vi "Lab Temp Monitor.vi"() -> ()   [LabVIEW 2012]
uses:
  Automated Dish Machine/LabVIEW/ADM2 - QMH Layout/support/Message Queue/Message Cluster.ctl
  <vilib>/Utility/error.llb/DialogType.ctl
  Automated Dish Machine/LabVIEW/ADM2 - QMH Layout/support/Message Queue/Message Queue.lvlib
panel:
  out "Limits":dbl[](array[numeric])
  in  "STOP":bool
  in  "Channel Names":string[](array[string])=["One", "Two", "Three", "Four", "Five", "Six"]
  out "Test Display":string
  in  "CONFIG":bool
  in  "Limit 1":dbl=52.0
  in  "Limit 2":dbl=56.0
  out "Timers":u32[](array[numeric])=[1, 95] format="%<%H:%M:%S>t"
  in  "Email / Image Rate":u32=7200 format="%<%H:%M:%S>t"
  in  "Graph / Log Rate":u32=2 format="%<%H:%M:%S>t"
  in  "START":bool
  in  "MAIN TAB":enum32{"Page 1", "Page 2"}(tab)
  out "Graph":cluster{"t0":dbl, "dx":dbl, "Y Values":dbl[][]}(graph)
  out "Email Error":errorcluster
  out "UI ERROR":errorcluster
  out "DAQ Error":errorcluster
  in  "9213 Config":T1={"Sample Rate [Hz]"=100.0, "Samples/Ch"=1, "Ch Used"=1, "Rolling Average"=1, "HI/LO Trim [%]"=1.0, "Sample Timing Engine"=2} {"Ch Used" min=1 max=16 step=1; "Sample Timing Engine" max=2; "Sample Rate [Hz]" min=0.0001 max=100.0 format="%#_6p"; "Samples/Ch" min=1 step=1; "Rolling Average" min=1 step=1; "HI/LO Trim [%]" min=1.0 max=99.0}
  in  "9213 Name":tag="cDAQ2Mod1"
  out "9213 Error":errorcluster
  in  "Image File Path":path=path "C:/Users/ottinbr/Documents/Projects/John Bolduc/Lab Temp Monitor/a.jpg"
  in  "Log Folder Path":path=path "C:/Users/ottinbr/Documents/Projects/John Bolduc/Lab Temp Monitor/a.jpg"
  out "MAIN Queue":T2
  out "MAIN Loop":i32
  out "EVENT Loop":i32
  out "DAQ Queue":T2
  out "DAQ Loop":i32
  out "Last Sent Time":timestamp format="%<%I:%M:%S %p\n%x>T"
  out "Image Error":errorcluster
  in  "EMAIL":bool
  in  "EXIT PROGRAM":bool
  in  "ECOLAB BUTTON":bool=TRUE
  out "Measurements":dbl[](array[numeric]) format="%.2f"
  # "F&B Lab Temp. Monitor"
  # "SETPOINT"
  # "ELAPSED"
  # "Temp Limits"
  # "Created by Blake Otting  June 2013"
  # "Last Updated 7-11-13"
  # "HH:MM:SS"
  # "°C"
  # "HH:MM:SS"
  # "°C"
  # "9213 Configuration"
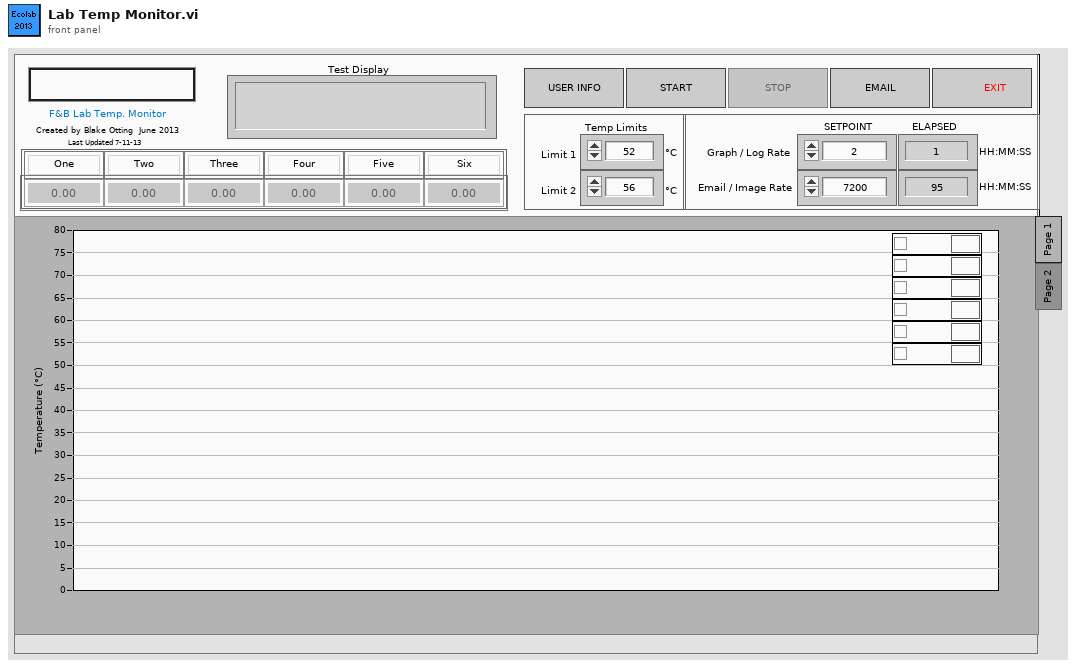
[diagram p1: front panel]
types:
  T1 = cluster{"Sample Rate [Hz]":dbl, "Samples/Ch":i32, "Ch Used":i32, "Rolling Average":i32, "HI/LO Trim [%]":dbl, "Sample Timing Engine":u32}
  T2 = cluster{"Message":string, "Message Data":variant}
  T3 = cluster{"Graph":cluster{"t0":dbl, "dx":dbl, "Y Values":dbl[][]}, "Image File Path":path, "Data Row":string[], "Log Folder Path":path, "Channel Names":string[], "Config":cluster{"First Name":string, "Last Name":string, "Alternate Email":string, "Test Name":string, "Test Description":string}, "Temp Limits":dbl[], "test running?":bool}
  T4 = cluster{"MAIN":refnum<queue>, "DAQ":refnum<queue>}
  T5 = typedef "Message Queue.lvlib/Message Cluster.ctl" = cluster{"Message":string, "Message Data":variant}
  T6 = typedef "DialogType.ctl" = u16
  T7 = cluster{"First Name":string, "Last Name":string, "Alternate Email":string, "Test Name":string, "Test Description":string}
  T8 = cluster{"CONFIG":enum8{"Enabled", "Disabled", "Disabled and Grayed Out"}, "START":enum8{"Enabled", "Disabled", "Disabled and Grayed Out"}, "STOP":enum8{"Enabled", "Disabled", "Disabled and Grayed Out"}, "EMAIL":enum8{"Enabled", "Disabled", "Disabled and Grayed Out"}}
  T9 = enum8{"Enabled", "Disabled", "Disabled and Grayed Out"}[]
  T10 = typedef "imagedata.ctl" = cluster{"image type":i32, "image depth":i32, "image":u8[], "mask":u8[], "colors":u32[], "Rectangle":cluster{"left":i16, "top":i16, "right":i16, "bottom":i16}}
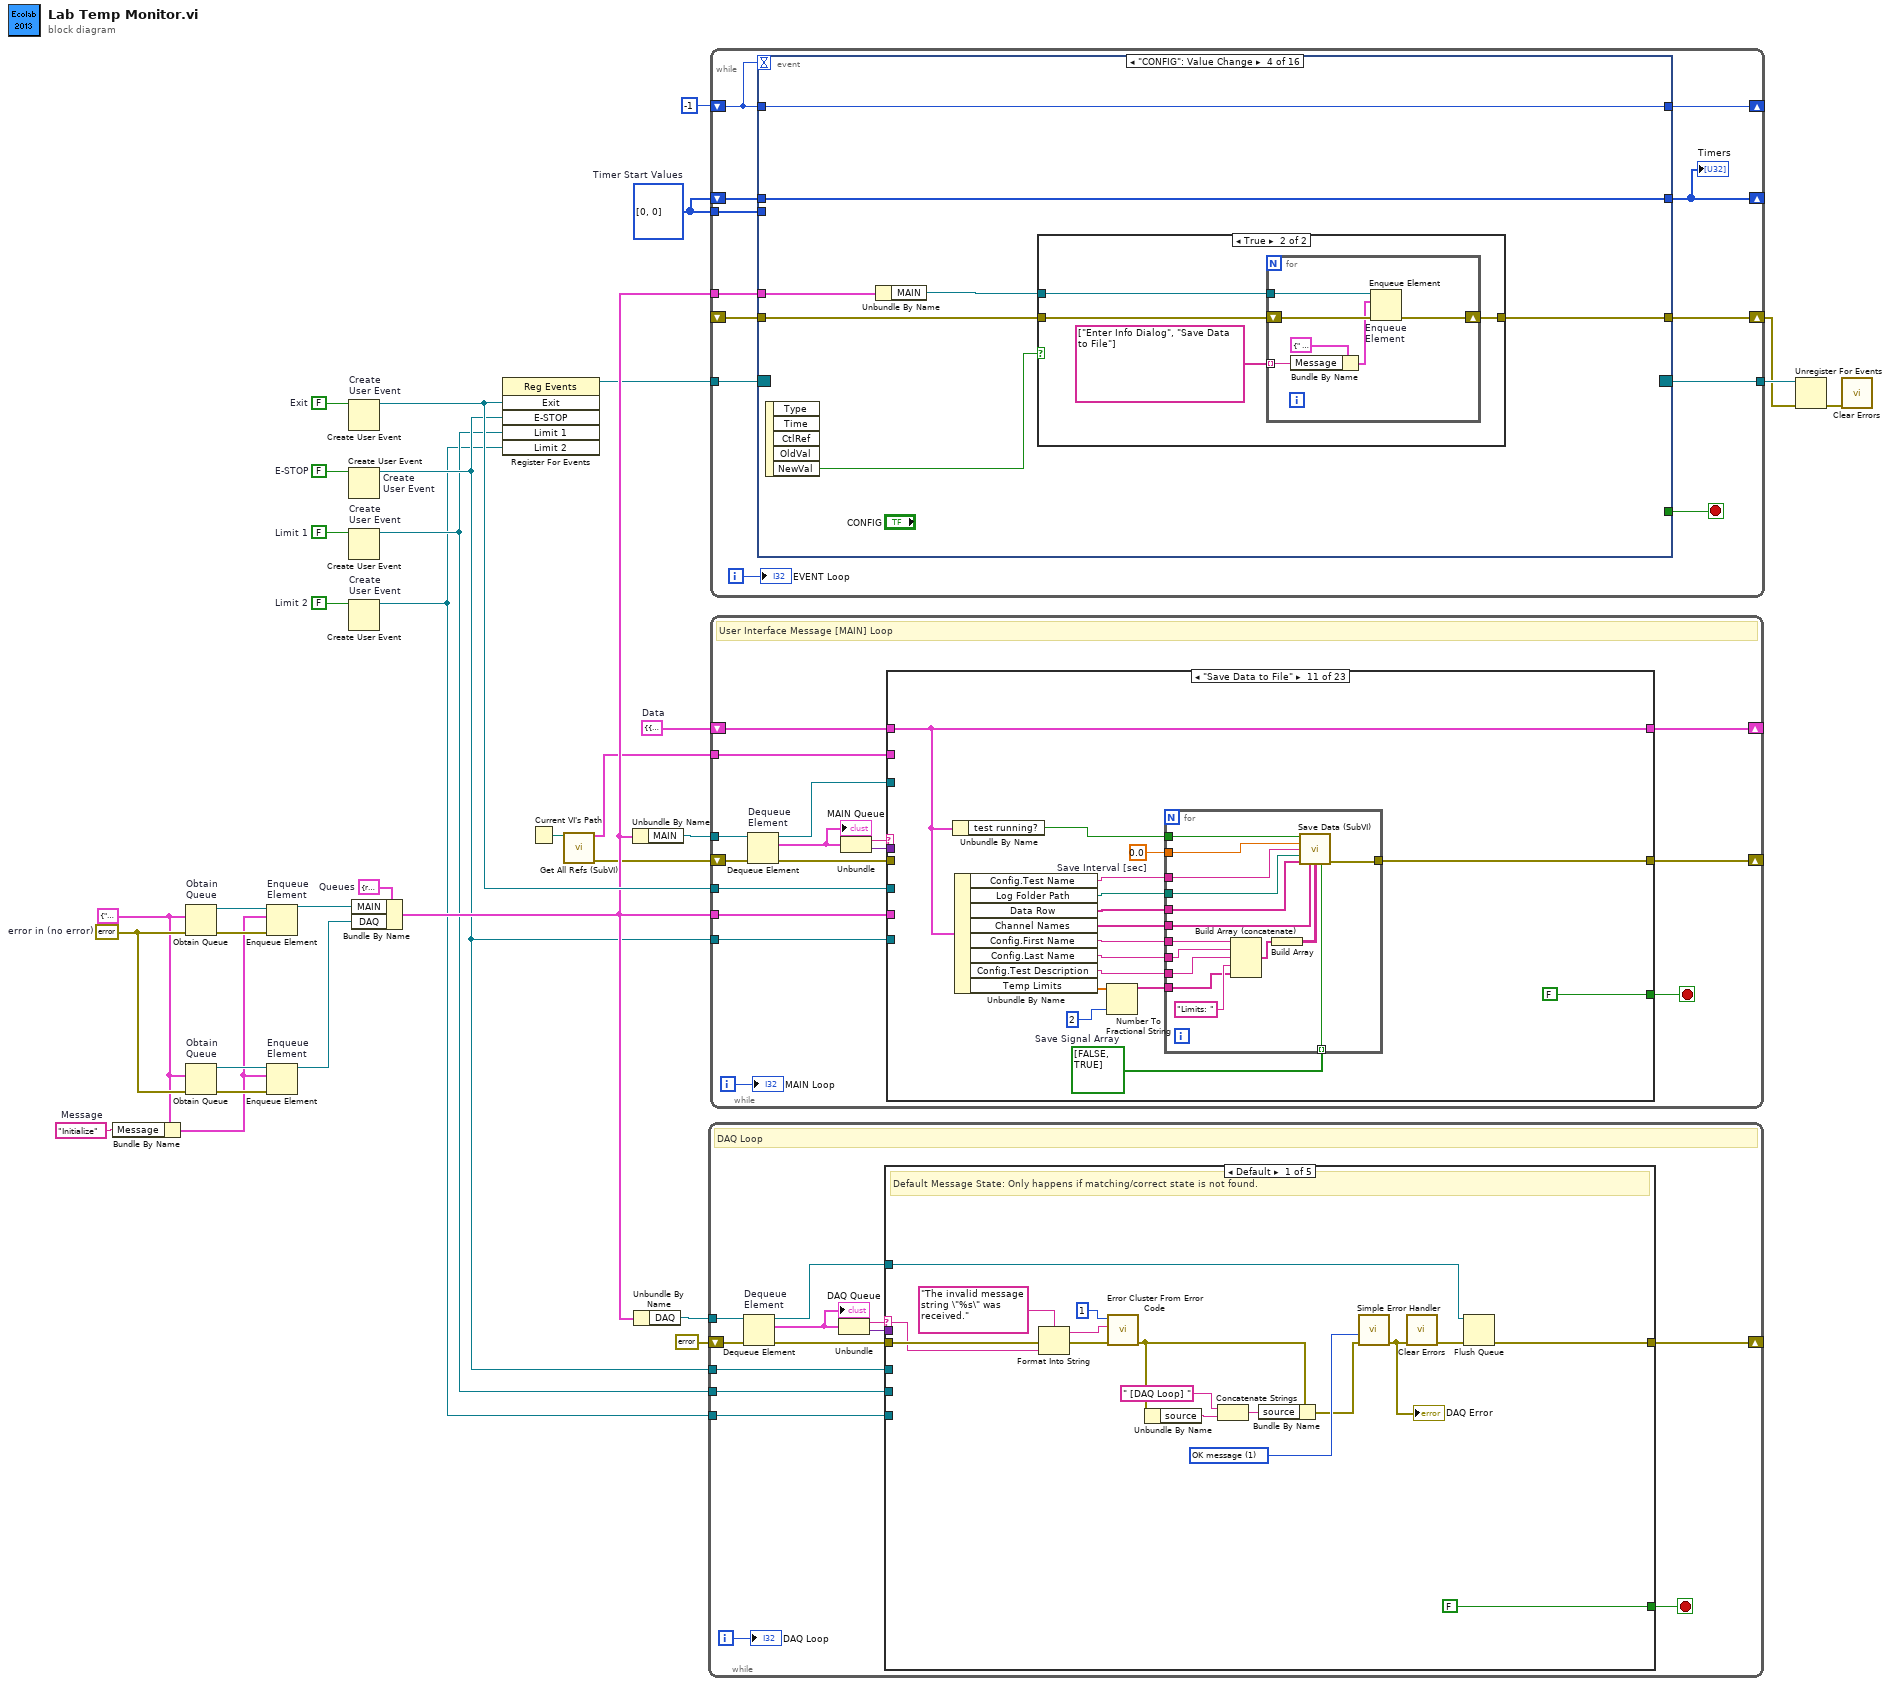
[diagram p0: block diagram]
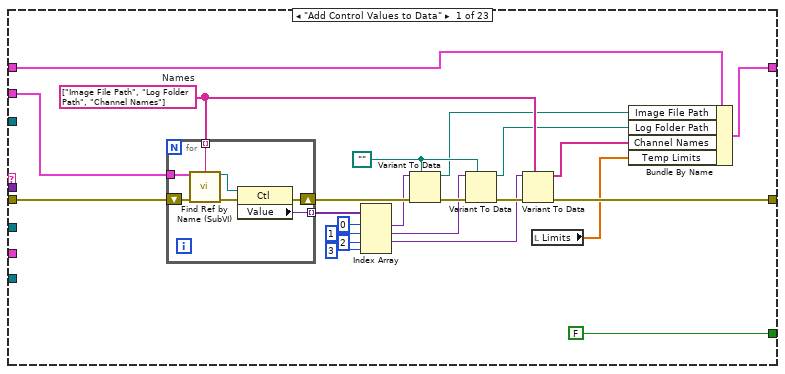
[diagram p2: hidden frame]
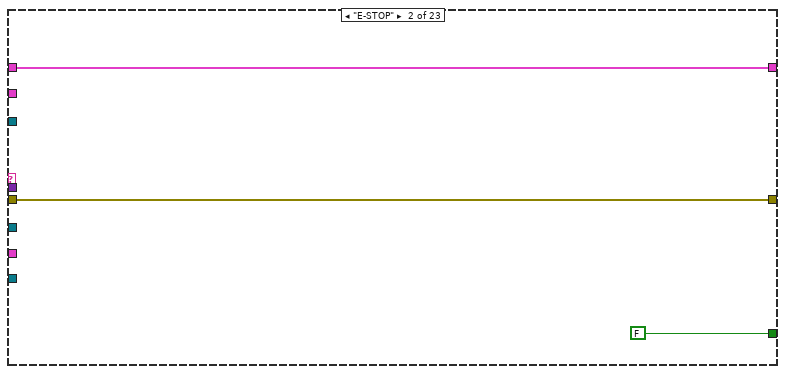
[diagram p3: hidden frame]
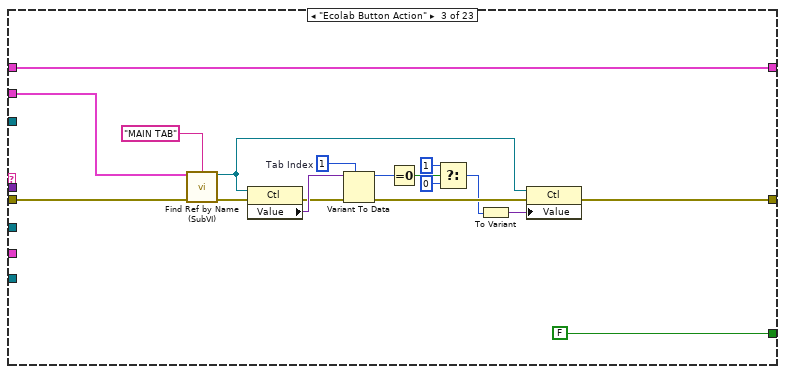
[diagram p4: hidden frame]
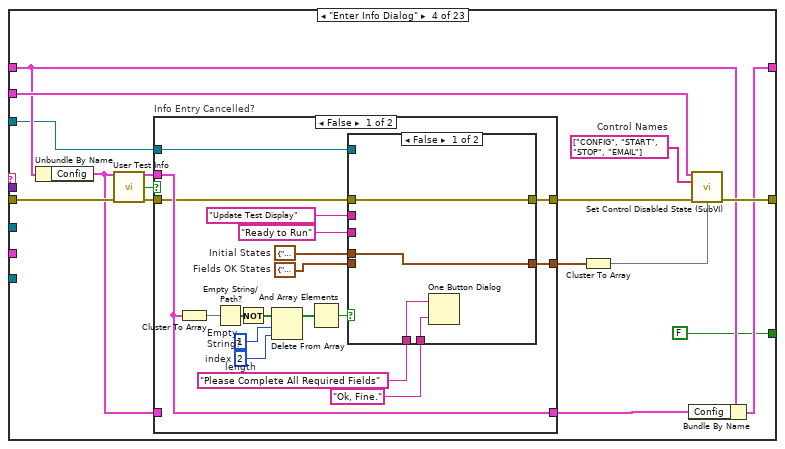
[diagram p5: hidden frame]
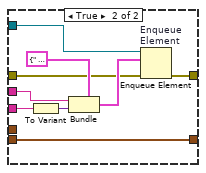
[diagram p6: hidden frame]
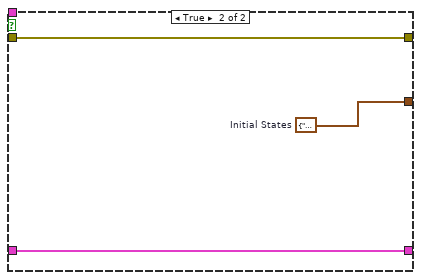
[diagram p7: hidden frame]
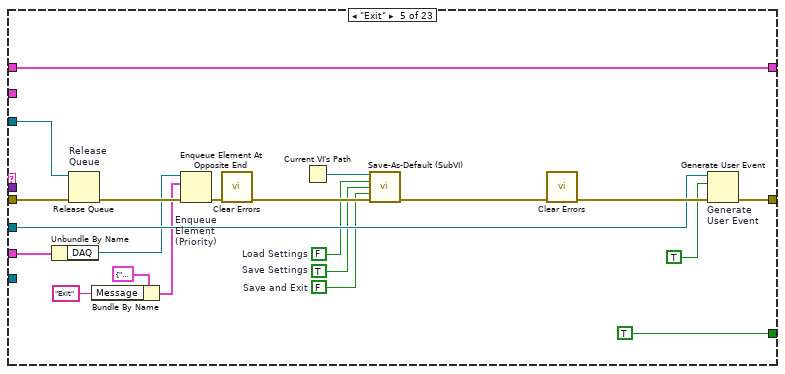
[diagram p8: hidden frame]
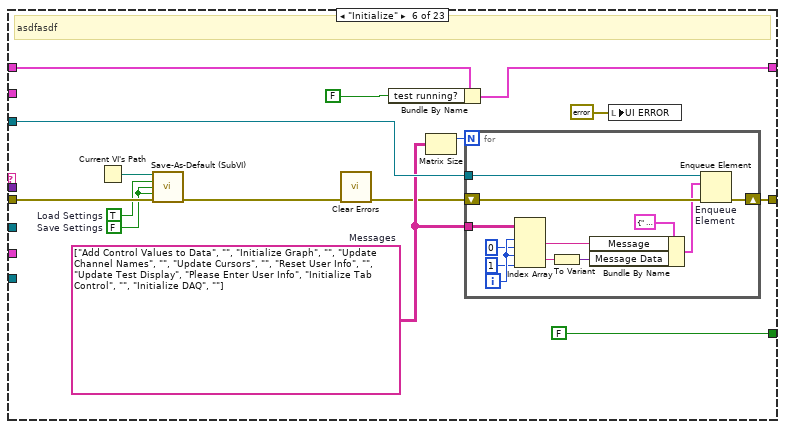
[diagram p9: hidden frame]
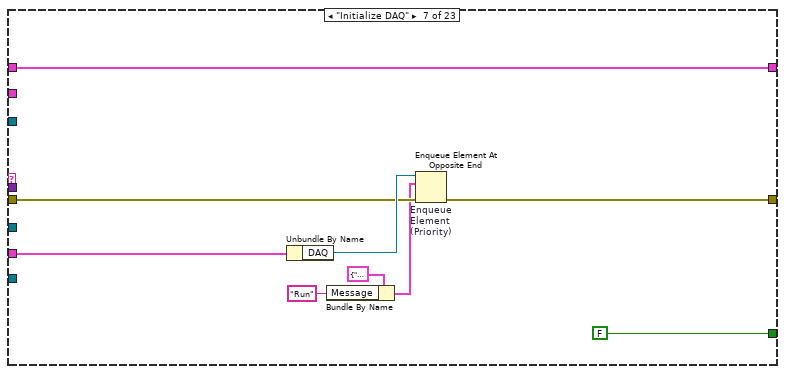
[diagram p10: hidden frame]
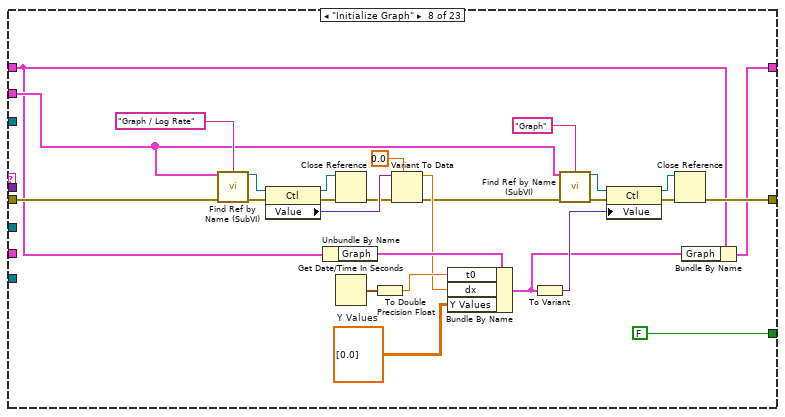
[diagram p11: hidden frame]
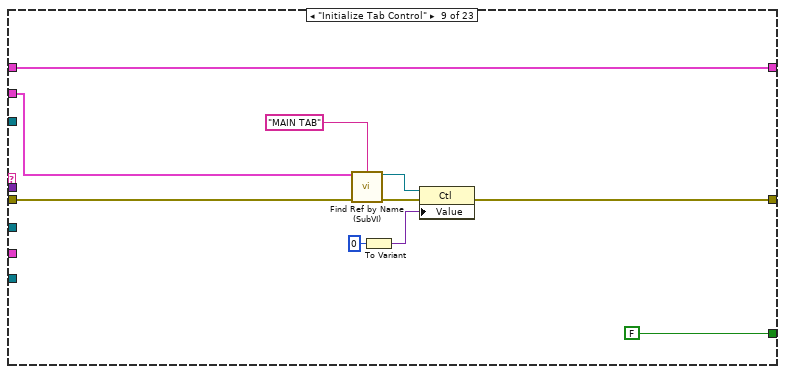
[diagram p12: hidden frame]
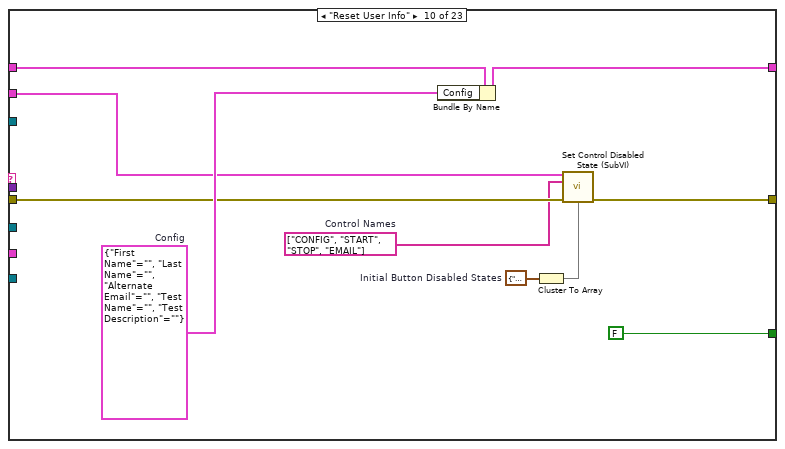
[diagram p13: hidden frame]
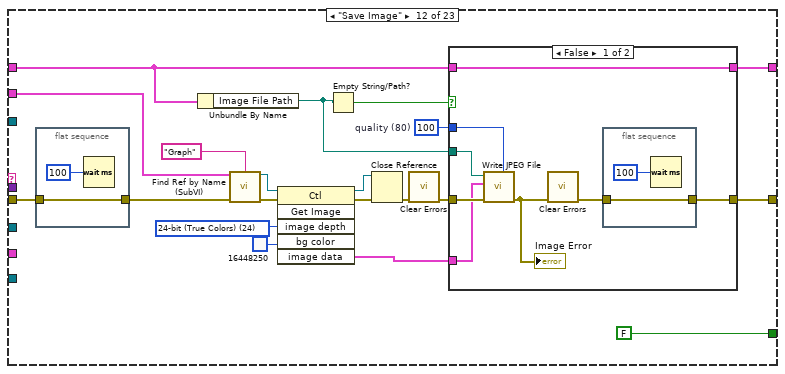
[diagram p14: hidden frame]
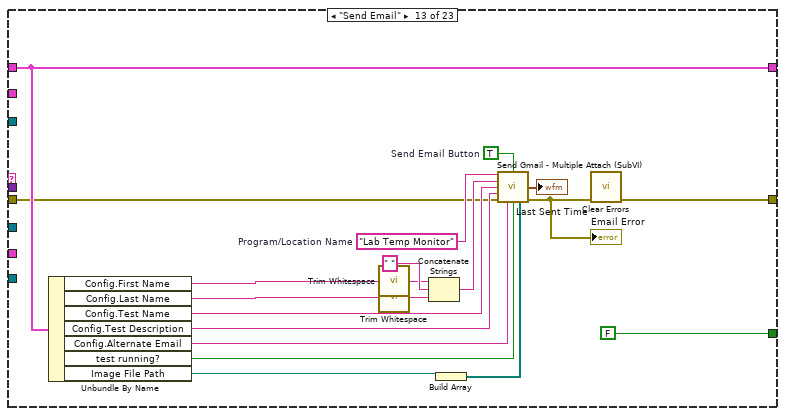
[diagram p16: hidden frame]
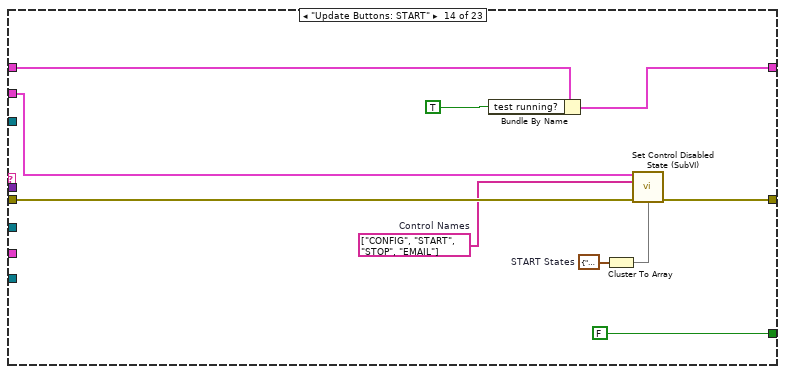
[diagram p17: hidden frame]
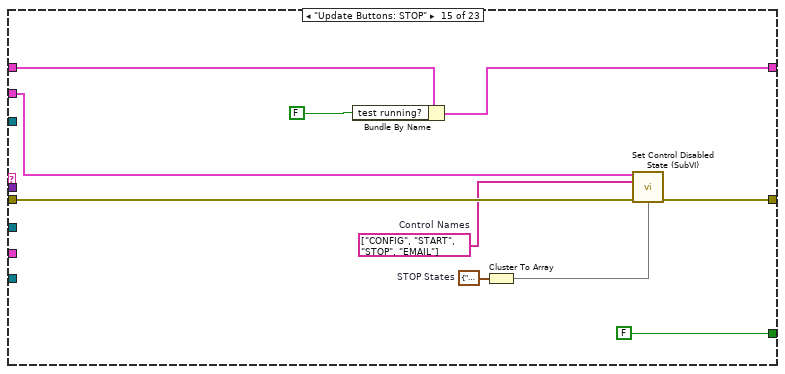
[diagram p18: hidden frame]
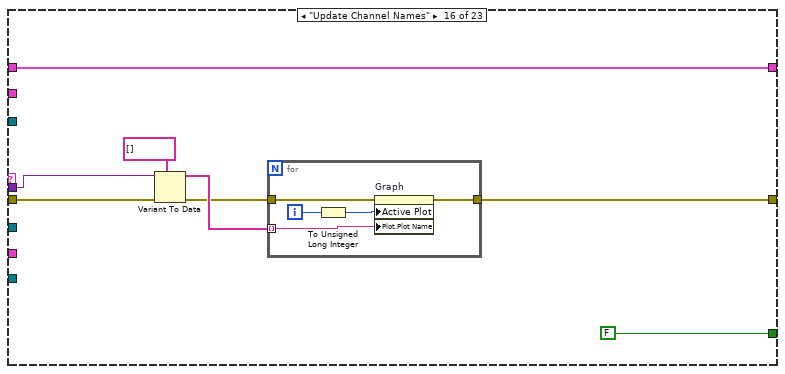
[diagram p19: hidden frame]
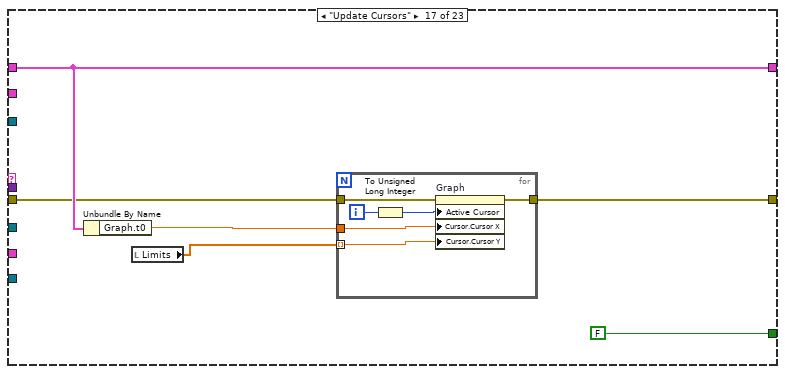
[diagram p20: hidden frame]
diagram:
  w5 = FALSE  # Limit 2
  w6 = FALSE  # Limit 1
  w28 = errorcluster {"status"=FALSE, "code"=0, "source"=""}  # error in (no error)
  w14 = FALSE  # E-STOP
  w7 = T3 {"Graph"={"t0"=0.0, "dx"=1.0, "Y Values"=[[0.0], [0.0], [0.0], [0.0], [0.0], [0.0]]}, "Image File Path"=path "", "Data Row"=[], "Log Folder Path"=path "", "Channel Names"=[], "Config"={"First Name"="", "Last Name"="", "Alternate Email"="", "Test Name"="", "Test Description"=""}, "Temp Limits"=[], "test running?"=FALSE}  # Data
  w18 = FALSE  # Exit
  w15 = u32[] [0, 0]  # Timer Start Values
  w25 = T4 {"MAIN"=refnum, "DAQ"=refnum}  # Queues
  w27 = T2 {"Message"="", "Message Data"=variant} ("Message Cluster")
  w33 = "Initialize"  # Message
  n1 = Bundle By Name(cluster=w27, "Message"=w33) -> (w26:T2)
  n2 = Obtain Queue "Obtain\nQueue"(element data type=w27, error in (no error)=w28) -> (queue out=w30:refnum<queue>, error out=w29:errorcluster)  [unwired: 3 in, 1 out]
  n3 = Obtain Queue "Obtain\nQueue"(element data type=w27, error in (no error)=w28) -> (queue out=w31:refnum<queue>, error out=w32:errorcluster)  [unwired: 3 in, 1 out]
  n4 = Enqueue Element "Enqueue\nElement"(queue=w30, element=w26, error in (no error)=w29) -> (queue out=w24:refnum<queue>)  [unwired: 1 in, 2 out]
  n5 = Enqueue Element "Enqueue\nElement"(queue=w31, element=w26, error in (no error)=w32) -> (queue out=w23:refnum<queue>)  [unwired: 1 in, 2 out]
  n6 = Create User Event "Create\nUser Event"(user event datatype=w18) -> (user event=w22:refnum<user-event>)  [unwired: 1 in, 1 out]
  n7 = Create User Event "Create\nUser Event"(user event datatype=w14) -> (user event=w13:refnum<user-event>)  [unwired: 1 in, 1 out]
  n8 = Create User Event "Create\nUser Event"(user event datatype=w6) -> (user event=w4:refnum<user-event>)  [unwired: 1 in, 1 out]
  n9 = Create User Event "Create\nUser Event"(user event datatype=w5) -> (user event=w3:refnum<user-event>)  [unwired: 1 in, 1 out]
  n10 = Bundle By Name(cluster=w25, "MAIN"=w24, "DAQ"=w23) -> (w20:T4)
  n11 = register-events(w22, w13, w4, w3) -> (reference out=w11:refnum<event-registration>)  [unwired: 2 in, 1 out]
  n12 = Current VI's Path() -> (path=w9:path)
  n13 = call "Get All Refs (SubVI).vi"("Current VI Path"=w9) -> ("Control Refs"=w8:cluster{"Label Name":string, "Ref":refnum<vi>}[], "Error OUT"=w10:errorcluster)  [unwired: 13 in]
  n14 = Unbundle By Name(w20) -> ("MAIN"=w16:refnum<queue>)
  n15 = Unbundle By Name(w20) -> ("DAQ"=w19:refnum<queue>)
  n16 = while {
    shift-right: [w44] -> _
    shift-left: errorcluster {"status"=FALSE, "code"=0, "source"=""} ("No Error") -> [w46]
    tunnel: w19 -> [w43]
    tunnel: w13 -> [w36]
    tunnel: w4 -> [w35]
    tunnel: w3 -> [w34]
    i -> [w37]
    stop <- w39 stop-if-true
    # "DAQ Loop"
    n17 = Dequeue Element "Dequeue\nElement"(queue=w43, error in (no error)=w46) -> (queue out=w45:refnum<queue>, element=w38:T5, error out=w42:errorcluster)  [unwired: 1 in, 1 out]
    "DAQ Queue" <- w38
    n18 = Unbundle(w38) -> ("Message"=w41:string, "Message Data"=w40:variant)
    n19 = case shown="Default" w41 {
      selector: w41 -> [w61 _ _ _ _]
      tunnel: w40 -> [_ _ _ _ _]
      tunnel: w42 -> [w62 w66 w71 w73 w111]
      tunnel: w45 -> [w49 _ w72 _ w106]
      tunnel: [w47 w65 w69 w73 w107] -> w44
      tunnel: [FALSE FALSE TRUE FALSE FALSE] -> w39
      tunnel: w36 -> [_ w64 _ _ _]
      tunnel: w35 -> [_ _ _ _ w97]
      tunnel: w34 -> [_ _ _ _ w94]
      frame Default {
        w56 = T6 1 items=["no dialog", "OK message", "continue or stop message", "OK message + warnings", "continue/stop + warnings"] ("type of dialog (OK msg:1)")
        # "Default Message State: Only happens if matching/correct state is not found."
        n20 = Format Into String(format string="The invalid message string \"%s\" was received." ("Invalid Message Loop Message"), error in=w62, w61) -> (resulting string=w58:string, error out=w57:errorcluster)  [unwired: 1 in]
        n21 = call <vilib>:"Error Cluster From Error Code.vi"("error in (no error)"=w57, "error message (\"\")"=w58, "error code (0)"=1) -> ("error out"=w55:errorcluster)  [unwired: 6 in]
        n22 = Unbundle By Name(w55) -> ("source"=w51:string)
        n23 = Concatenate Strings(" [DAQ Loop] " ("error source (\" \")"), w51) -> (w54:string)
        n24 = Bundle By Name(cluster=w55, "source"=w54) -> (w53:errorcluster)
        n25 = call <vilib>:"Simple Error Handler.vi"("type of dialog (OK msg:1)"=w56, "error in (no error)"=w53) -> ("error out"=w50:errorcluster)  [unwired: 3 in, 4 out]
        "DAQ Error" <- w50
        n26 = call <vilib>:"Clear Errors.vi"("error in (no error)"=w50) -> ("error out"=w48:errorcluster)  [unwired: 6 in]
        n27 = Flush Queue(queue=w49, error in (no error)=w48) -> (error out=w47:errorcluster)  [unwired: 2 out]
      }
      frame "E-STOP" {
        n28 = Generate User Event "Generate\nUser Event"(user event=w64, event data cluster=TRUE ("event data"), error in=w66) -> (error out=w65:errorcluster)  [unwired: 1 out]
      }
      frame "Exit" {
        n29 = Release Queue "Release\nQueue"(queue=w72, error in (no error)=w71) -> (error out=w69:errorcluster)  [unwired: 1 in, 2 out]
      }
      frame "Initialize" {
        # "Main Loop Initilizes DAQ to RUN"
        # "Clear DAQ Error"
        n30 = local write "DAQ Error"(errorcluster {"status"=FALSE, "code"=0, "source"=""} ("No Error")) -> ()
      }
      frame "Run" {
        w80 = 6  # # of Channels
        # "Convert\n°F to °C"
        # "Run Continuously Unless Error or Exit Message"
        n31 = Build Array("Limit 1", "Limit 2") -> (→"Limits":dbl[])
        n32 = call "DAQmx 9213 16ch K Thermocouple (SubVI).vi"("9213 Name"="9213 Name", "9213 Config"="9213 Config", "Error Input"=w111) -> ("Measurements"=w82:dbl[], "9213 Error"=w76:errorcluster)  [unwired: 11 in]
        "9213 Error" <- w76
        n33 = Subtract(x=w82, y=32.0) -> (x-y=w101:dbl[])
        n34 = Divide(x=w101, y=1.8) -> (x/y=w81:dbl[])
        n35 = Array Subset "Array\nSubset"(array=w81, index=0, length=w80) -> (→"Measurements":dbl[])
        n36 = Array Subset(array=w81, index=1, length=5) -> (w78:dbl[])
        n37 = Greater Or Equal?(x=w78, y="Limit 1") -> (x >= y?=w98:bool[])
        n38 = Greater Or Equal?(x=w78, y="Limit 2") -> (x >= y?=w93:bool[])
        n39 = Or Array Elements(Boolean array=w98) -> (logical OR=w89:bool)
        n40 = Or Array Elements(Boolean array=w93) -> (logical OR=w84:bool)
        n41 = feedback-in #1(w89) -> ()
        n42 = feedback #1() -> (w90:bool)  [unwired: 1 in]
        n43 = feedback #2() -> (w86:bool)  [unwired: 1 in]
        n44 = feedback-in #2(w84) -> ()
        n45 = Not Equal?(x=w89, y=w90) -> (x != y?=w88:bool)
        n46 = Not Equal?(x=w84, y=w86) -> (x != y?=w85:bool)
        n47 = And(x=w89, y=w88) -> (x .and. y?=w87:bool)
        n48 = And(x=w84, y=w85) -> (x .and. y?=w83:bool)
        n49 = case shown="True" w87 {
          tunnel: w76 -> [w119 w123]
          tunnel: [w119 w122] -> w96
          tunnel: w97 -> [_ w120]
          frame False {
          }
          frame True {
            n50 = Generate User Event "Generate\nUser Event"(user event=w120, event data cluster=TRUE ("event data"), error in=w123) -> (error out=w122:errorcluster)  [unwired: 1 out]
          }
        }
        n51 = case shown="True" w83 {
          tunnel: w96 -> [w114 w118]
          tunnel: [w114 w117] -> w95
          tunnel: w94 -> [_ w115]
          frame False {
          }
          frame True {
            n52 = Generate User Event "Generate\nUser Event"(user event=w115, event data cluster=TRUE ("event data"), error in=w118) -> (error out=w117:errorcluster)  [unwired: 1 out]
          }
        }
        n53 = Bundle By Name(cluster=T2 {"Message"="", "Message Data"=variant} ("Message Cluster"), "Message"="Run") -> (w108:T2)
        n54 = Enqueue Element "Enqueue\nElement"(queue=w106, element=w108, error in (no error)=w95) -> (error out=w107:errorcluster)  [unwired: 1 in, 2 out]
      }
    }
    "DAQ Loop" <- w37
  }
  n55 = while {
    tunnel: w11 -> [w134]
    shift-right: [w132] -> _
    shift-left: -1 -> [w133]
    shift-right: [w126] -> _
    shift-left: w15 -> [w131]
    tunnel: w20 -> [w130]
    shift-right: [w129] -> w2
    shift-left: _ -> [w128]
    tunnel: w15 -> [w125]
    tunnel: [w124] -> w12
    i -> [w127]
    stop <- w135 stop-if-true
    n56 = event shown="[3] \"CONFIG\": Value Change" {
      selector: w134 -> [_ _ _ _ _ _ _ _ _ _ _ _ _ _ _ _]
      dyn-events: [_ _ _ _ _ _ _ _ _ _ _ _ _ _ _ _] -> w124
      timeout: w133 -> [_ _ _ _ _ _ _ _ _ _ _ _ _ _ _ _]
      tunnel: [FALSE _ _ _ _ _ _ FALSE w298 w301 _ _ _ _ _ _] -> w135
      tunnel: w133 -> [w153 _ _ w234 w246 w274 w285 w297 w299 w303 w321 w323 w332 w340 w355 w358]
      tunnel: [w153 w190 w212 w234 w246 w274 w285 w297 w299 w303 w321 w323 w332 w340 w355 w358] -> w132
      tunnel: w131 -> [w152 _ _ w233 w247 w273 w284 w286 w300 w302 w320 w322 w331 w341 w356 w357]
      tunnel: [w150 w191 w211 w233 w247 w273 w284 w286 w300 w302 w320 w322 w331 w341 w356 w357] -> w126
      tunnel: w130 -> [w151 w186 w208 w229 w249 w265 w276 w292 _ w306 w316 _ w326 w336 w352 w363]
      tunnel: [w149 w187 w207 w230 w250 w267 w278 w290 _ w304 w313 _ w324 w337 w345 w361] -> w129
      tunnel: w128 -> [w145 w188 w209 w231 w251 w268 w279 w293 _ w305 w317 _ w325 w338 w353 w362]
      tunnel: w125 -> [_ w191 w211 _ _ _ _ _ _ _ _ _ _ _ _ _]
      event Timeout {
        w140 = string[] ["Save Image", "Send Email"]  # Email Messages
        w139 = string[] ["Update Graph", "Save Data to File", "Update Cursors"]  # Graph / Log Messages
        n57 = event-data() -> ()  [unwired: 1 in, 2 out]
        n58 = Increment "Increment\n(1 Second)"(x=w152) -> (x+1=w144:u32[])
        n59 = Unbundle By Name "Queue"(w151) -> ("MAIN"=w146:refnum<queue>)
        n60 = Build Array("Graph / Log Rate", "Email / Image Rate") -> (w147:u32[])
        n61 = Build Array(w139, w140) -> (w148:string[][])
        n62 = Array Size(array=w139) -> (size(s)=w138:i32)
        n63 = Array Size(array=w140) -> (size(s)=w137:i32)
        n64 = Build Array(w138, w137) -> (w136:i32[])
        n65 = for {
          tunnel: w146 -> [w161]
          shift-right: [w160] -> w149
          shift-left: w145 -> [w159]
          tunnel: w148 -> [w157] mode=indexing
          tunnel: w147 -> [w156] mode=indexing
          shift-right: [w162] -> w150
          shift-left: w144 -> [w155]
          tunnel: w136 -> [w154] mode=indexing
          i -> [w158]
          n66 = in-place {
            in-place-border: w157 -> [w168]
            in-place-border: [w167] -> w160
            in-place-border: w161 -> [w166]
            in-place-border: w159 -> [w165]
            in-place-border: w156 -> [w164]
            in-place-border: w154 -> [w163]
            n67 = in-place-array #3(w155, w158) -> (w171:u32)
            n68 = Greater Or Equal? ("Seconds\nElapsed?")(x=w171, y=w164) -> (x >= y?=w169:bool)
            n69 = case shown="True" w169 {
              tunnel: w171 -> [w173 _]
              tunnel: [w173 u32 0] -> w170
              tunnel: w168 -> [_ w178]
              tunnel: [w172 w175] -> w167
              tunnel: w166 -> [_ w177]
              tunnel: w165 -> [w172 w176]
              tunnel: w163 -> [_ w174]
              frame False {
              }
              frame True {
                # "Time Elapsed"
                n70 = for {
                  N: w174 -> [_]
                  tunnel: w178 -> [w180] mode=indexing
                  tunnel: w177 -> [w185]
                  shift-right: [w184] -> w175
                  shift-left: w176 -> [w183]
                  n71 = Bundle By Name(cluster=T2 {"Message"="", "Message Data"=variant} ("Message Cluster"), "Message"=w180) -> (w181:T2)
                  n72 = Enqueue Element "Enqueue\nElement"(queue=w185, element=w181, error in (no error)=w183) -> (error out=w184:errorcluster)  [unwired: 1 in, 2 out]
                }
              }
            }
            n73 = in-place-array #3(w170) -> (w162:u32[])  [unwired: 1 out]
          }
        }
      }
      event "START": Value Change {
        w190 = 1000  # milliseconds
        # "1 Second \"Stopwatch\" Timer Value"
        n74 = event-data() -> ("NewVal"=w189:bool)  [unwired: 1 in, 4 out]
        n75 = case shown="True" w189 {
          tunnel: w188 -> [w192 w196]
          tunnel: [w192 w197] -> w187
          tunnel: w186 -> [_ w195]
          frame False {
          }
          frame True {
            w193 = string[] ["Not used", "Test Running", "Not Used"]  # Message Data
            w198 = string[] ["Initialize Graph", "Update Test Display", "Update Buttons: START"]  # Messages
            n76 = Unbundle By Name(w195) -> ("MAIN"=w194:refnum<queue>)
            n77 = for {
              shift-right: [w206] -> w197
              shift-left: w196 -> [w205]
              tunnel: w198 -> [w202] mode=indexing
              tunnel: w194 -> [w203]
              tunnel: w193 -> [w200] mode=indexing
              n78 = To Variant(anything=w200) -> (Variant=w199:variant)
              n79 = Bundle By Name(cluster=T2 {"Message"=" ", "Message Data"=variant} ("Message Cluster"), "Message"=w202, "Message Data"=w199) -> (w204:T2)
              n80 = Enqueue Element "Enqueue\nElement"(queue=w203, element=w204, error in (no error)=w205) -> (error out=w206:errorcluster)  [unwired: 1 in, 2 out]
            }
          }
        }
      }
      event "STOP": Value Change {
        w212 = -1  # Stop Timers by not having Timeout
        n81 = event-data() -> ("NewVal"=w210:bool)  [unwired: 1 in, 4 out]
        n82 = case shown="True" w210 {
          tunnel: w209 -> [w213 w217]
          tunnel: [w213 w218] -> w207
          tunnel: w208 -> [_ w216]
          frame False {
          }
          frame True {
            w214 = string[] ["Test Stopped", "Not Used"]  # Message Data
            w219 = string[] ["Update Test Display", "Update Buttons: STOP"]  # Messages
            n83 = Unbundle By Name(w216) -> ("MAIN"=w215:refnum<queue>)
            n84 = for {
              shift-right: [w227] -> w218
              shift-left: w217 -> [w226]
              tunnel: w219 -> [w223] mode=indexing
              tunnel: w215 -> [w224]
              tunnel: w214 -> [w221] mode=indexing
              n85 = To Variant(anything=w221) -> (Variant=w220:variant)
              n86 = Bundle By Name(cluster=T2 {"Message"=" ", "Message Data"=variant} ("Message Cluster"), "Message"=w223, "Message Data"=w220) -> (w225:T2)
              n87 = Enqueue Element "Enqueue\nElement"(queue=w224, element=w225, error in (no error)=w226) -> (error out=w227:errorcluster)  [unwired: 1 in, 2 out]
            }
          }
        }
      }
      event "CONFIG": Value Change {
        n88 = event-data() -> ("NewVal"=w232:bool)  [unwired: 1 in, 4 out]
        n89 = Unbundle By Name(w229) -> ("MAIN"=w228:refnum<queue>)
        n90 = case shown="True" w232 {
          tunnel: w231 -> [w235 w236]
          tunnel: [w235 w237] -> w230
          tunnel: w228 -> [_ w239]
          frame False {
          }
          frame True {
            n91 = for {
              shift-right: [w245] -> w237
              shift-left: w236 -> [w244]
              tunnel: string[] ["Enter Info Dialog", "Save Data to File"] -> [w240] mode=indexing
              tunnel: w239 -> [w241]
              n92 = Bundle By Name(cluster=T2 {"Message"=" ", "Message Data"=variant} ("Message Cluster"), "Message"=w240) -> (w242:T2)
              n93 = Enqueue Element "Enqueue\nElement"(queue=w241, element=w242, error in (no error)=w244) -> (error out=w245:errorcluster)  [unwired: 1 in, 2 out]
            }
          }
        }
      }
      event "EMAIL": Value Change {
        n94 = event-data() -> ("NewVal"=w248:bool)  [unwired: 1 in, 4 out]
        n95 = case shown="False" w248 {
          tunnel: w251 -> [w259 w263]
          tunnel: [w255 w263] -> w250
          tunnel: w249 -> [w258 _]
          frame False {
            w254 = T2 {"Message"="", "Message Data"=variant} ("Message Cluster")
            n96 = Bundle By Name(cluster=w254, "Message"="Save Image") -> (w260:T2)
            n97 = Unbundle By Name(w258) -> ("MAIN"=w261:refnum<queue>)
            n98 = Enqueue Element "Enqueue\nElement"(queue=w261, element=w260, error in (no error)=w259) -> (queue out=w256:refnum<queue>, error out=w257:errorcluster)  [unwired: 1 in, 1 out]
            n99 = Bundle By Name(cluster=w254, "Message"="Send Email") -> (w252:T2)
            n100 = Enqueue Element "Enqueue\nElement"(queue=w256, element=w252, error in (no error)=w257) -> (error out=w255:errorcluster)  [unwired: 1 in, 2 out]
          }
          frame True {
          }
        }
      }
      event "Image File Path": Value Change {
        n101 = event-data() -> ()  [unwired: 1 in, 5 out]
        n102 = To Variant(anything="Image File Path") -> (Variant=w266:variant)
        n103 = Bundle By Name(cluster=T2 {"Message"="", "Message Data"=variant} ("Message Cluster"), "Message"="Update Image Path", "Message Data"=w266) -> (w270:T2)
        n104 = Unbundle By Name(w265) -> ("MAIN"=w271:refnum<queue>)
        n105 = Enqueue Element "Enqueue\nElement"(queue=w271, element=w270, error in (no error)=w268) -> (error out=w267:errorcluster)  [unwired: 1 in, 2 out]
      }
      event "Log Folder Path": Value Change {
        n106 = event-data() -> ()  [unwired: 1 in, 5 out]
        n107 = To Variant(anything="Log Folder Path") -> (Variant=w277:variant)
        n108 = Bundle By Name(cluster=T2 {"Message"="", "Message Data"=variant} ("Message Cluster"), "Message"="Update Log Path", "Message Data"=w277) -> (w281:T2)
        n109 = Unbundle By Name(w276) -> ("MAIN"=w282:refnum<queue>)
        n110 = Enqueue Element "Enqueue\nElement"(queue=w282, element=w281, error in (no error)=w279) -> (error out=w278:errorcluster)  [unwired: 1 in, 2 out]
      }
      event "EXIT PROGRAM": Value Change {
        n111 = event-data() -> ()  [unwired: 1 in, 5 out]
        n112 = Unbundle By Name(w292) -> ("MAIN"=w294:refnum<queue>)
        n113 = Unbundle By Name(w292) -> ("DAQ"=w288:refnum<queue>)
        n114 = Bundle By Name(cluster=T2 {"Message"="", "Message Data"=variant} ("Message Cluster"), "Message"="Exit") -> (w289:T2)
        n115 = Enqueue Element At Opposite End "Enqueue\nElement\n(Priority)"(queue=w294, element=w289, error in (no error)=w293) -> (error out=w291:errorcluster)  [unwired: 1 in, 2 out]
        n116 = Enqueue Element At Opposite End "Enqueue\nElement\n(Priority)"(queue=w288, element=w289, error in (no error)=w291) -> (error out=w290:errorcluster)  [unwired: 1 in, 2 out]
      }
      event User Event {
        # "All Loops Stopped?"
        n117 = event-data() -> ("Exit"=w298:bool)  [unwired: 1 in, 3 out]
      }
      event User Event {
        w301 = FALSE  # Exit
        n118 = event-data() -> ()  [unwired: 1 in, 4 out]
        n119 = Unbundle By Name(w306) -> ("MAIN"=w310:refnum<queue>)
        n120 = Unbundle By Name(w306) -> ("DAQ"=w307:refnum<queue>)
        n121 = Bundle By Name(cluster=T2 {"Message"="", "Message Data"=variant} ("Message Cluster"), "Message"="Exit") -> (w308:T2)
        n122 = Enqueue Element At Opposite End "Enqueue\nElement\n(Priority)"(queue=w310, element=w308, error in (no error)=w305) -> (error out=w309:errorcluster)  [unwired: 1 in, 2 out]
        n123 = Enqueue Element At Opposite End "Enqueue\nElement\n(Priority)"(queue=w307, element=w308, error in (no error)=w309) -> (error out=w304:errorcluster)  [unwired: 1 in, 2 out]
      }
      event User Event {
        n124 = event-data() -> ()  [unwired: 1 in, 4 out]
        n125 = Unbundle By Name(w316) -> ("MAIN"=w315:refnum<queue>)
        n126 = Bundle By Name(cluster=T2 {"Message"="", "Message Data"=variant} ("Message Cluster"), "Message"="Send Email") -> (w314:T2)
        n127 = Enqueue Element At Opposite End "Enqueue\nElement\n(Priority)"(queue=w315, element=w314, error in (no error)=w317) -> (error out=w313:errorcluster)  [unwired: 1 in, 2 out]
      }
      event User Event {
        n128 = event-data() -> ()  [unwired: 1 in, 4 out]
      }
      event "ECOLAB BUTTON": Value Change {
        n129 = event-data() -> ()  [unwired: 1 in, 5 out]
        n130 = Bundle By Name(cluster=T2 {"Message"="", "Message Data"=variant} ("Message Cluster"), "Message"="Ecolab Button Action") -> (w328:T2)
        n131 = Unbundle By Name(w326) -> ("MAIN"=w329:refnum<queue>)
        n132 = Enqueue Element "Enqueue\nElement"(queue=w329, element=w328, error in (no error)=w325) -> (error out=w324:errorcluster)  [unwired: 1 in, 2 out]
      }
      event "Limit 1", "Limit 2": Value Change; "Graph": Cursor Move {
        n133 = event-data() -> ()  [unwired: 1 in, 3 out]
        n134 = Bundle By Name(cluster=T2 {"Message"="", "Message Data"=variant} ("Message Cluster"), "Message"="Update Cursors") -> (w334:T2)
        n135 = Unbundle By Name(w336) -> ("MAIN"=w335:refnum<queue>)
        n136 = Enqueue Element "Enqueue\nElement"(queue=w335, element=w334, error in (no error)=w338) -> (error out=w337:errorcluster)  [unwired: 1 in, 2 out]
      }
      event "Channel Names": Value Change {
        w343 = T2 {"Message"="", "Message Data"=variant} ("Message Cluster")
        n137 = event-data() -> ()  [unwired: 1 in, 5 out]
        n138 = To Variant(anything="Channel Names") -> (Variant=w349:variant)
        n139 = Bundle By Name(cluster=w343, "Message"="Update Channel Names", "Message Data"=w349) -> (w350:T2)
        n140 = Unbundle By Name(w352) -> ("MAIN"=w351:refnum<queue>)
        n141 = Enqueue Element "Enqueue\nElement"(queue=w351, element=w350, error in (no error)=w353) -> (queue out=w347:refnum<queue>, error out=w346:errorcluster)  [unwired: 1 in, 1 out]
        n142 = Bundle By Name(cluster=w343, "Message"="Save Data to File") -> (w342:T2)
        n143 = Enqueue Element "Enqueue\nElement"(queue=w347, element=w342, error in (no error)=w346) -> (error out=w345:errorcluster)  [unwired: 1 in, 2 out]
      }
      event "Graph / Log Rate": Value Change {
        n144 = event-data() -> ("NewVal"=w360:u32)  [unwired: 1 in, 4 out]
        n145 = To Variant(anything=w360) -> (Variant=w359:variant)
        n146 = Bundle By Name(cluster=T2 {"Message"="", "Message Data"=variant} ("Message Cluster"), "Message"="Update Graph Interval", "Message Data"=w359) -> (w365:T2)
        n147 = Unbundle By Name(w363) -> ("MAIN"=w366:refnum<queue>)
        n148 = Enqueue Element "Enqueue\nElement"(queue=w366, element=w365, error in (no error)=w362) -> (error out=w361:errorcluster)  [unwired: 1 in, 2 out]
      }
    }
    "Timers" <- w126
    "EVENT Loop" <- w127
  }
  n149 = while {
    shift-right: [w381] -> _
    shift-left: w10 -> [w383]
    tunnel: w16 -> [w371]
    tunnel: w20 -> [w380]
    tunnel: w22 -> [w375]
    shift-right: [w373] -> _
    shift-left: w7 -> [w374]
    tunnel: w13 -> [w369]
    tunnel: w8 -> [w368]
    i -> [w372]
    stop <- w370 stop-if-true
    # "User Interface Message [MAIN] Loop"
    n150 = Dequeue Element "Dequeue\nElement"(queue=w371, error in (no error)=w383) -> (queue out=w382:refnum<queue>, element=w376:T5, error out=w379:errorcluster)  [unwired: 1 in, 1 out]
    "MAIN Queue" <- w376
    n151 = Unbundle(w376) -> ("Message"=w378:string, "Message Data"=w377:variant)
    n152 = case shown="\"Save Data to File\"" w378 {
      selector: w378 -> [_ _ _ _ _ _ _ _ _ _ _ _ _ _ _ _ _ _ _ _ _ _ w780]
      tunnel: w377 -> [_ _ _ _ _ _ _ _ _ _ _ _ _ _ _ w699 _ _ w736 w743 w751 w763 _]
      tunnel: w379 -> [w400 w416 w434 w450 w504 w519 w538 w554 w577 w585 _ w622 w654 w680 w690 w698 w709 w719 w733 w744 w752 w762 w781]
      tunnel: w382 -> [_ _ _ w436 w505 w513 _ _ _ _ _ _ _ _ _ _ _ _ _ _ _ _ w772]
      tunnel: [w386 w416 w433 w443 w502 w514 w537 w556 w575 w584 w604 w629 w672 w679 w689 w696 w711 w719 w732 w740 w748 w761 w775] -> w381
      tunnel: w380 -> [_ _ _ _ w499 _ w536 _ _ _ _ _ _ _ _ _ _ _ _ _ _ _ _]
      tunnel: [FALSE FALSE FALSE FALSE TRUE FALSE FALSE FALSE FALSE FALSE FALSE FALSE FALSE FALSE FALSE FALSE FALSE FALSE FALSE FALSE FALSE FALSE FALSE] -> w370
      tunnel: w375 -> [_ _ _ _ w493 _ _ _ _ _ _ _ _ _ _ _ _ _ _ _ _ _ _]
      tunnel: w374 -> [w388 w414 w430 w437 w485 w508 w534 w546 w570 w588 w590 w636 w655 w675 w685 w695 w712 w722 w738 w746 w754 w758 w777]
      tunnel: [w406 w414 w430 w438 w485 w507 w534 w544 w570 w587 w590 w635 w655 w674 w684 w695 w712 w721 w737 w741 w749 w757 w777] -> w373
      tunnel: w369 -> [_ _ _ _ _ _ _ _ _ _ _ _ _ _ _ _ _ _ _ _ _ _ w773]
      tunnel: w368 -> [w405 _ w431 w442 _ _ _ w547 w574 w581 _ w631 _ w681 w691 _ _ _ _ _ _ _ _]
      frame "Add Control Values to Data" {
        w392 = string[] ["Image File Path", "Log Folder Path", "Channel Names"]  # Names
        w393 = path ""
        n153 = for {
          tunnel: w405 -> [w411]
          tunnel: w392 -> [w410] mode=indexing
          tunnel: [w407] -> w404 mode=indexing
          shift-right: [w409] -> w399
          shift-left: w400 -> [w408]
          n154 = call "Find Ref by Name (SubVI).vi"("Control Refs"=w411, "Label Name"=w410, "Error IN"=w408) -> ("Control Reference"=w413:refnum<vi>, "Error OUT"=w412:errorcluster)  [unwired: 11 in]
          n155 = property class="Ctl"(reference=w413, error in=w412) -> (error out=w409:errorcluster, "Value"=w407:variant)  [unwired: 1 out]
        }
        n156 = Index Array(array=w404, index #1=0, index #2=1, index #3=2, index #4=3) -> (element #1=w396:variant, element #2=w395:variant, element #3=w394:variant)  [unwired: 1 out]
        n157 = Variant To Data(error in=w399, type=w393, Variant=w396) -> (data=w389:path, error out=w398:errorcluster)
        n158 = Variant To Data(error in=w398, type=w393, Variant=w395) -> (data=w390:path, error out=w397:errorcluster)
        n159 = Variant To Data(error in=w397, type=w392, Variant=w394) -> (data=w391:string[], error out=w386:errorcluster)
        n160 = local read "Limits"() -> (w385:dbl[])
        n161 = Bundle By Name(cluster=w388, "Image File Path"=w389, "Log Folder Path"=w390, "Channel Names"=w391, "Temp Limits"=w385) -> (w406:T3)
      }
      frame "E-STOP" {
      }
      frame "Ecolab Button Action" {
        w427 = u32 1  # Tab Index
        n162 = call "Find Ref by Name (SubVI).vi"("Control Refs"=w431, "Label Name"="MAIN TAB", "Error IN"=w434) -> ("Control Reference"=w424:refnum<vi>, "Error OUT"=w428:errorcluster)  [unwired: 11 in]
        n163 = property class="Ctl"(reference=w424, error in=w428) -> (error out=w425:errorcluster, "Value"=w426:variant)  [unwired: 1 out]
        n164 = Variant To Data(error in=w425, type=w427, Variant=w426) -> (data=w422:u32, error out=w423:errorcluster)
        n165 = Equal To 0?(x=w422) -> (x = 0?=w421:bool)
        n166 = Select(t=u32 1, s=w421, f=u32 0) -> (s? t:f=w418:u32)
        n167 = To Variant(anything=w418) -> (Variant=w429:variant)
        n168 = property class="Ctl"(reference=w424, error in=w423, "Value"=w429) -> (error out=w433:errorcluster)  [unwired: 1 out]
      }
      frame "Enter Info Dialog" {
        w441 = string[] ["CONFIG", "START", "STOP", "EMAIL"]  # Control Names
        n169 = Unbundle By Name(w437) -> ("Config"=w448:T7)
        n170 = call "User Test Info.vi"("CONFIG IN"=w448, "Error IN"=w450) -> ("CONFIG OUT"=w446:T7, "Cancelled?"=w449:bool, "Error OUT"=w445:errorcluster)  [unwired: 11 in]
        n171 = case "Info Entry Cancelled?" shown="False" w449 {
          tunnel: w448 -> [_ w484]
          tunnel: [w468 w484] -> w447
          tunnel: w446 -> [w468 _]
          tunnel: w445 -> [w453 w483]
          tunnel: [w452 w483] -> w444
          tunnel: [w456 w482] -> w439
          tunnel: w436 -> [w454 _]
          frame False {
            w458 = T8 {"CONFIG"=enum."Enabled", "START"=enum."Enabled", "STOP"=enum."Disabled and Grayed Out", "EMAIL"=enum."Enabled"}  # Fields OK States
            w457 = T8 {"CONFIG"=enum."Enabled", "START"=enum."Disabled and Grayed Out", "STOP"=enum."Disabled and Grayed Out", "EMAIL"=enum."Disabled and Grayed Out"}  # Initial States
            w464 = 1  # length
            w465 = 2  # index
            n172 = Cluster To Array(cluster=w468) -> (array=w467:string[])
            n173 = Empty String/Path? "Empty\nString?"(string/path=w467) -> (empty?=w466:bool[])
            n174 = Not(x=w466) -> (.not. x?=w463:bool[])
            n175 = Delete From Array ("Delete \nAlt. Email Add.\nFrom Array")(array=w463, length=w464, index=w465) -> (array with subset deleted=w462:bool[])  [unwired: 1 out]
            n176 = And Array Elements(Boolean array=w462) -> (logical AND=w461:bool)
            n177 = case shown="False" w461 {
              tunnel: "Please Complete All Required Fields" ("message") -> [w472 _]
              tunnel: "Ok, Fine." ("button name (\"OK\")") -> [w471 _]
              tunnel: w458 -> [_ w481]
              tunnel: w457 -> [w470 _]
              tunnel: [w470 w481] -> w456
              tunnel: "Update Test Display" ("Message") -> [_ w477]
              tunnel: w454 -> [_ w476]
              tunnel: w453 -> [w469 w475]
              tunnel: [w469 w474] -> w452
              tunnel: "Ready to Run" -> [_ w473]
              frame False {
                n178 = One Button Dialog(message=w472, button name ("OK")=w471) -> ()  [unwired: 1 out]
              }
              frame True {
                n179 = To Variant(anything=w473) -> (Variant=w478:variant)
                n180 = Bundle(cluster=T2 {"Message"=" ", "Message Data"=variant} ("Message Cluster"), "Message"=w477, "Message Data"=w478) -> (w479:T2)
                n181 = Enqueue Element "Enqueue\nElement"(queue=w476, element=w479, error in (no error)=w475) -> (error out=w474:errorcluster)  [unwired: 1 in, 2 out]
              }
            }
          }
          frame True {
            w482 = T8 {"CONFIG"=enum."Enabled", "START"=enum."Disabled and Grayed Out", "STOP"=enum."Disabled and Grayed Out", "EMAIL"=enum."Disabled and Grayed Out"}  # Initial States
          }
        }
        n182 = Cluster To Array(cluster=w439) -> (array=w440:T9)
        n183 = Bundle By Name(cluster=w437, "Config"=w447) -> (w438:T3)
        n184 = call "Set Control Disabled State (SubVI).vi"("Control Refs"=w442, "Control Names"=w441, "Error IN"=w444, "Disable Status"=w440) -> ("Error OUT"=w443:errorcluster)  [unwired: 11 in]
      }
      frame "Exit" {
        w492 = FALSE  # Save and Exit
        w490 = TRUE  # Save Settings
        w491 = FALSE  # Load Settings
        n185 = Unbundle By Name(w499) -> ("DAQ"=w487:refnum<queue>)
        n186 = Release Queue "Release\nQueue"(queue=w505, error in (no error)=w504) -> (error out=w497:errorcluster)  [unwired: 1 in, 2 out]
        n187 = Bundle By Name(cluster=T2 {"Message"="", "Message Data"=variant} ("Message Cluster"), "Message"="Exit") -> (w488:T2)
        n188 = Enqueue Element At Opposite End "Enqueue\nElement\n(Priority)"(queue=w487, element=w488, error in (no error)=w497) -> (error out=w500:errorcluster)  [unwired: 1 in, 2 out]
        n189 = call <vilib>:"Clear Errors.vi"("error in (no error)"=w500) -> ("error out"=w496:errorcluster)  [unwired: 6 in]
        n190 = Current VI's Path() -> (path=w489:path)
        n191 = call "Save-As-Default (SubVI).vi"("Current VI's Path"=w489, "Load Settings"=w491, "Save Settings"=w490, "Save and Exit"=w492, "Error IN"=w496) -> ("Save as Default Error"=w495:errorcluster)  [unwired: 10 in]
        n192 = call <vilib>:"Clear Errors.vi"("error in (no error)"=w495) -> ("error out"=w494:errorcluster)  [unwired: 6 in]
        n193 = Generate User Event "Generate\nUser Event"(user event=w493, event data cluster=TRUE ("event data"), error in=w494) -> (error out=w502:errorcluster)  [unwired: 1 out]
      }
      frame "Initialize" {
        w512 = string[][] [["Add Control Values to Data", ""], ["Initialize Graph", ""], ["Update Channel Names", ""], ["Update Cursors", ""], ["Reset User Info", ""], ["Update Test Display", "Please Enter User Info"], ["Initialize Tab Control", ""], ["Initialize DAQ", ""]]  # Messages
        w517 = FALSE  # Save Settings
        w518 = TRUE  # Load Settings
        # "asdfasdf"
        n194 = Current VI's Path() -> (path=w516:path)
        n195 = call "Save-As-Default (SubVI).vi"("Current VI's Path"=w516, "Load Settings"=w518, "Save Settings"=w517, "Save and Exit"=w517, "Error IN"=w519) -> ("Save as Default Error"=w509:errorcluster)  [unwired: 10 in]
        n196 = call <vilib>:"Clear Errors.vi"("error in (no error)"=w509) -> ("error out"=w510:errorcluster)  [unwired: 6 in]
        n197 = Bundle By Name(cluster=w508, "test running?"=FALSE) -> (w507:T3)
        n198 = Matrix Size(0:w512) -> (1:w511:i32)  [unwired: 1 out]
        n199 = for {
          N: w511 -> [_]
          shift-right: [w532] -> w514
          shift-left: w510 -> [w531]
          tunnel: w513 -> [w529]
          tunnel: w512 -> [w527]
          i -> [w524]
          n200 = Index Array(array=w527, index (row) #1=w524, index (col) #1=0, index (row) #2=w524, index (col) #2=1) -> (element #1=w521:string, element #2=w526:string)
          n201 = To Variant(anything=w526) -> (Variant=w525:variant)
          n202 = Bundle By Name(cluster=T2 {"Message"=" ", "Message Data"=variant} ("Message Cluster"), "Message"=w521, "Message Data"=w525) -> (w530:T2)
          n203 = Enqueue Element "Enqueue\nElement"(queue=w529, element=w530, error in (no error)=w531) -> (error out=w532:errorcluster)  [unwired: 1 in, 2 out]
        }
        n204 = local write "UI ERROR"(errorcluster {"status"=FALSE, "code"=0, "source"=""} ("No Error")) -> ()
      }
      frame "Initialize DAQ" {
        n205 = Unbundle By Name(w536) -> ("DAQ"=w539:refnum<queue>)
        n206 = Bundle By Name(cluster=T2 {"Message"="", "Message Data"=variant} ("Message Cluster"), "Message"="Run") -> (w535:T2)
        n207 = Enqueue Element At Opposite End "Enqueue\nElement\n(Priority)"(queue=w539, element=w535, error in (no error)=w538) -> (error out=w537:errorcluster)  [unwired: 1 in, 2 out]
      }
      frame "Initialize Graph" {
        w543 = dbl[][] [[0.0]]  # Y Values
        n208 = call "Find Ref by Name (SubVI).vi"("Control Refs"=w547, "Label Name"="Graph / Log Rate", "Error IN"=w554) -> ("Control Reference"=w553:refnum<vi>, "Error OUT"=w552:errorcluster)  [unwired: 11 in]
        n209 = property class="Ctl"(reference=w553, error in=w552) -> (reference out=w564:refnum<vi>, error out=w565:errorcluster, "Value"=w566:variant)
        n210 = Unbundle By Name(w546) -> ("Graph"=w562:cluster{"t0":dbl, "dx":dbl, "Y Values":dbl[][]})
        n211 = Close Reference(reference=w564, error in (no error)=w565) -> (error out=w563:errorcluster)
        n212 = Get Date/Time In Seconds() -> (seconds since 1Jan1904=w568:timestamp)
        n213 = To Double Precision Float(number=w568) -> (double precision float=w561:dbl)
        n214 = Variant To Data(error in=w563, type=0.0, Variant=w566) -> (data=w559:dbl, error out=w551:errorcluster)
        n215 = Bundle By Name(cluster=w562, "t0"=w561, "dx"=w559, "Y Values"=w543) -> (w545:cluster{"t0":dbl, "dx":dbl, "Y Values":dbl[][]})
        n216 = To Variant(anything=w545) -> (Variant=w560:variant)
        n217 = call "Find Ref by Name (SubVI).vi"("Control Refs"=w547, "Label Name"="Graph", "Error IN"=w551) -> ("Control Reference"=w558:refnum<vi>, "Error OUT"=w550:errorcluster)  [unwired: 11 in]
        n218 = property class="Ctl"(reference=w558, error in=w550, "Value"=w560) -> (reference out=w555:refnum<vi>, error out=w557:errorcluster)
        n219 = Close Reference(reference=w555, error in (no error)=w557) -> (error out=w556:errorcluster)
        n220 = Bundle By Name(cluster=w546, "Graph"=w545) -> (w544:T3)
      }
      frame "Initialize Tab Control" {
        n221 = call "Find Ref by Name (SubVI).vi"("Control Refs"=w574, "Label Name"="MAIN TAB", "Error IN"=w577) -> ("Control Reference"=w573:refnum<vi>, "Error OUT"=w576:errorcluster)  [unwired: 11 in]
        n222 = To Variant(anything=0) -> (Variant=w572:variant)
        n223 = property class="Ctl"(reference=w573, error in=w576, "Value"=w572) -> (error out=w575:errorcluster)  [unwired: 1 out]
      }
      frame "Reset User Info" {
        w580 = string[] ["CONFIG", "START", "STOP", "EMAIL"]  # Control Names
        w583 = T8 {"CONFIG"=enum."Enabled", "START"=enum."Disabled and Grayed Out", "STOP"=enum."Disabled and Grayed Out", "EMAIL"=enum."Disabled and Grayed Out"}  # Initial Button Disabled States
        w586 = T7 {"First Name"="", "Last Name"="", "Alternate Email"="", "Test Name"="", "Test Description"=""}  # Config
        n224 = Bundle By Name(cluster=w588, "Config"=w586) -> (w587:T3)
        n225 = Cluster To Array(cluster=w583) -> (array=w582:T9)
        n226 = call "Set Control Disabled State (SubVI).vi"("Control Refs"=w581, "Control Names"=w580, "Error IN"=w585, "Disable Status"=w582) -> ("Error OUT"=w584:errorcluster)  [unwired: 11 in]
      }
      frame "Save Data to File" {
        w601 = bool[] [FALSE, TRUE]  # Save Signal Array
        w603 = 0.0  # Save Interval [sec]
        n227 = Unbundle By Name(w590) -> ("test running?"=w589:bool)
        n228 = Unbundle By Name(w590) -> ("Config.Test Name"=w602:string, "Log Folder Path"=w600:path, "Data Row"=w599:string[], "Channel Names"=w598:string[], "Config.First Name"=w595:string, "Config.Last Name"=w594:string, "Config.Test Description"=w593:string, "Temp Limits"=w591:dbl[])
        n229 = Number To Fractional String(number=w591, precision (6)=i16 2) -> (F-format string=w592:string[])  [unwired: 2 in]
        n230 = for {
          tunnel: [w619] -> w604
          tunnel: w589 -> [w618]
          tunnel: w603 -> [w617]
          tunnel: w602 -> [w616]
          tunnel: w601 -> [w615] mode=indexing
          tunnel: w599 -> [w614]
          tunnel: w600 -> [w613]
          tunnel: w598 -> [w612]
          tunnel: w595 -> [w611]
          tunnel: w594 -> [w608]
          tunnel: w593 -> [w607]
          tunnel: w592 -> [w605]
          n231 = Build Array (concatenate)(w611, w608, w607, "Limits: ", w605) -> (w610:string[])
          n232 = Build Array(w610) -> (w609:string[][])
          n233 = call "Save Data (SubVI).vi"("Save Enable"=w618, "Save Interval [sec]"=w617, "File Name"=w616, "Folder Location"=w613, "Data Array (Row)"=w614, "Column Header Array"=w612, "Title Block"=w609, "External Save Signal"=w615) -> ("Save Error"=w619:errorcluster)  [unwired: 5 in, 2 out]
        }
      }
      frame "Save Image" {
        w630 = 100  # quality (80)
        w637 = u16 24 items=["1-bit (Black and White)"=1, "4-bit (16 colors)"=4, "8-bit (256 colors)"=8, "24-bit (True Colors)"=24] ("Image Color Depth")
        n234 = flat-sequence {
          tunnel: w622 -> [w640]
          tunnel: [w640] -> w621
          frame #0 {
            n235 = Wait (ms)(milliseconds to wait=u32 100) -> ()  [unwired: 1 out]
          }
        }
        n236 = Unbundle By Name(w636) -> ("Image File Path"=w628:path)
        n237 = call "Find Ref by Name (SubVI).vi"("Control Refs"=w631, "Label Name"="Graph", "Error IN"=w621) -> ("Control Reference"=w633:refnum<vi>, "Error OUT"=w634:errorcluster)  [unwired: 11 in]
        n238 = invoke class="Ctl" method="Get Image"(reference=w633, error in=w634, "image depth"=w637, "bg color"=u32 16448250) -> (reference out=w625:refnum<vi>, error out=w624:errorcluster, "image data"=w639:T10)  [unwired: 2 in, 3 out]
        n239 = Empty String/Path?(string/path=w628) -> (empty?=w627:bool)
        n240 = Close Reference(reference=w625, error in (no error)=w624) -> (error out=w623:errorcluster)
        n241 = call <vilib>:"Clear Errors.vi"("error in (no error)"=w623) -> ("error out"=w620:errorcluster)  [unwired: 6 in]
        n242 = case shown="False" w627 {
          tunnel: w620 -> [w649 w652]
          tunnel: w639 -> [w648 _]
          tunnel: w636 -> [w645 w653]
          tunnel: [w645 w653] -> w635
          tunnel: w630 -> [w647 _]
          tunnel: [w643 w652] -> w629
          tunnel: w628 -> [w646 _]
          frame False {
            n243 = call <vilib>:"Write JPEG File.vi"("quality (80)"=w647, "error in (no error)"=w649, "image data"=w648, "path to JPEG file"=w646) -> ("error out"=w644:errorcluster)  [unwired: 6 in, 1 out]
            "Image Error" <- w644
            n244 = call <vilib>:"Clear Errors.vi"("error in (no error)"=w644) -> ("error out"=w642:errorcluster)  [unwired: 6 in]
            n245 = flat-sequence {
              tunnel: w642 -> [w650]
              tunnel: [w650] -> w643
              frame #0 {
                n246 = Wait (ms)(milliseconds to wait=u32 100) -> ()  [unwired: 1 out]
              }
            }
          }
          frame True {
          }
        }
      }
      frame "Send Email" {
        w658 = TRUE  # Send Email Button
        w664 = "Lab Temp Monitor"  # Program/Location Name
        n247 = Unbundle By Name(w655) -> ("Config.First Name"=w668:string, "Config.Last Name"=w667:string, "Config.Test Name"=w661:string, "Config.Test Description"=w660:string, "Config.Alternate Email"=w657:string, "test running?"=w659:bool, "Image File Path"=w656:path)
        n248 = call <vilib>:"Trim Whitespace.vi"("string"=w668) -> ("trimmed string"=w669:string)  [unwired: 1 in]
        n249 = call <vilib>:"Trim Whitespace.vi"("string"=w667) -> ("trimmed string"=w671:string)  [unwired: 1 in]
        n250 = Concatenate Strings(w669, " ", w671) -> (w663:string)
        n251 = Build Array(w656) -> (w662:path[])
        n252 = call "Send Gmail - Multiple Attach (SubVI).vi"("Program/Location Name"=w664, "Send Email Button"=w658, "Test Operator (First Last)"=w663, "Test Name (Subject)"=w661, "Test Description (Body)"=w660, "Error IN"=w654, "Alternate Email"=w657, "Send Email Signal (Event)"=w659, "Attachment Path(s)"=w662) -> ("Last Sent Time"=→"Last Sent Time":timestamp, "Email Error"=w666:errorcluster)  [unwired: 4 in, 1 out]
        "Email Error" <- w666
        n253 = call <vilib>:"Clear Errors.vi"("error in (no error)"=w666) -> ("error out"=w672:errorcluster)  [unwired: 6 in]
      }
      frame "Update Buttons: START" {
        w678 = string[] ["CONFIG", "START", "STOP", "EMAIL"]  # Control Names
        w683 = T8 {"CONFIG"=enum."Disabled and Grayed Out", "START"=enum."Disabled and Grayed Out", "STOP"=enum."Enabled", "EMAIL"=enum."Enabled"}  # START States
        n254 = Bundle By Name(cluster=w675, "test running?"=TRUE) -> (w674:T3)
        n255 = Cluster To Array(cluster=w683) -> (array=w682:T9)
        n256 = call "Set Control Disabled State (SubVI).vi"("Control Refs"=w681, "Control Names"=w678, "Error IN"=w680, "Disable Status"=w682) -> ("Error OUT"=w679:errorcluster)  [unwired: 11 in]
      }
      frame "Update Buttons: STOP" {
        w688 = string[] ["CONFIG", "START", "STOP", "EMAIL"]  # Control Names
        w693 = T8 {"CONFIG"=enum."Enabled", "START"=enum."Enabled", "STOP"=enum."Disabled and Grayed Out", "EMAIL"=enum."Enabled"}  # STOP States
        n257 = Bundle By Name(cluster=w685, "test running?"=FALSE) -> (w684:T3)
        n258 = Cluster To Array(cluster=w693) -> (array=w692:T9)
        n259 = call "Set Control Disabled State (SubVI).vi"("Control Refs"=w691, "Control Names"=w688, "Error IN"=w690, "Disable Status"=w692) -> ("Error OUT"=w689:errorcluster)  [unwired: 11 in]
      }
      frame "Update Channel Names" {
        n260 = Variant To Data(error in=w698, type=string[] [], Variant=w699) -> (data=w700:string[], error out=w697:errorcluster)
        n261 = for {
          tunnel: w700 -> [w704] mode=indexing
          tunnel: w697 -> [w703]
          tunnel: [w702] -> w696
          i -> [w706]
          n262 = To Unsigned Long Integer(number=w706) -> (unsigned 32bit integer=w705:u32)
          n263 = property on="Graph" class="WFGraph (strict)"(error in=w703, "Active Plot"=w705, "Plot.Plot Name"=w704) -> (error out=w702:errorcluster)  [unwired: 1 in, 1 out]
        }
      }
      frame "Update Cursors" {
        n264 = Unbundle By Name(w712) -> ("Graph.t0"=w708:dbl)
        n265 = local read "Limits"() -> (w707:dbl[])
        n266 = for {
          tunnel: w707 -> [w715] mode=indexing
          tunnel: w708 -> [w716]
          tunnel: w709 -> [w714]
          tunnel: [w713] -> w711
          i -> [w718]
          n267 = To Unsigned Long Integer(number=w718) -> (unsigned 32bit integer=w717:u32)
          n268 = property on="Graph" class="WFGraph (strict)"(error in=w714, "Active Cursor"=w717, "Cursor.Cursor X"=w716, "Cursor.Cursor Y"=w715) -> (error out=w713:errorcluster)  [unwired: 1 in, 1 out]
        }
      }
      frame "Update Graph" {
        n269 = in-place {
          n270 = in-place-cluster #4(w722) -> ("Graph.Y Values"=w730:dbl[][])  [unwired: 1 out]
          n271 = local read "Measurements"() -> (w724:dbl[])
          n272 = Transpose 2D Array "Transpose"(2D array=w730) -> (transposed array=w728:dbl[][])
          n273 = Build Array (concatenate)(w728, w724) -> (w729:dbl[][])
          n274 = Transpose 2D Array "Transpose"(2D array=w729) -> (transposed array=w727:dbl[][])
          n275 = Number To Fractional String(number=w724, precision (6)=i16 1) -> (F-format string=w726:string[])  [unwired: 2 in]
          n276 = in-place-cluster #4("Graph.Y Values"=w727, "Data Row"=w726) -> (w721:T3)
        }
        n277 = Unbundle By Name(w721) -> ("Graph"=→"Graph":cluster{"t0":dbl, "dx":dbl, "Y Values":dbl[][]})
      }
      frame "Update Graph Interval" {
        n278 = Variant To Data(error in=w733, type=0.0, Variant=w736) -> (data=w734:dbl, error out=w732:errorcluster)
        n279 = Bundle By Name(cluster=w738, "Graph.dx"=w734) -> (w737:T3)
      }
      frame "Update Image Path" {
        n280 = Variant To Data(error in=w744, type=path "", Variant=w743) -> (data=w742:path, error out=w740:errorcluster)
        n281 = Bundle By Name(cluster=w746, "Image File Path"=w742) -> (w741:T3)
      }
      frame "Update Log Path" {
        n282 = Variant To Data(error in=w752, type=path "", Variant=w751) -> (data=w750:path, error out=w748:errorcluster)
        n283 = Bundle By Name(cluster=w754, "Log Folder Path"=w750) -> (w749:T3)
      }
      frame "Update Test Display" {
        n284 = Variant To Data(error in=w762, type="", Variant=w763) -> (data=w759:string, error out=w761:errorcluster)
        "Test Display" <- w759
        n285 = Equal?(x=w759, y="Test Running") -> (x = y?=w756:bool)
        n286 = Bundle By Name(cluster=w758, "test running?"=w756) -> (w757:T3)
      }
      frame Default {
        w776 = TRUE  # E-STOP
        # "Default Message State: Matching State Not Found or Error"
        n287 = Format Into String(format string="The invalid message string \"%s\" was received." ("Invalid Message Loop Message"), error in=w781, w780) -> (resulting string=w782:string, error out=w779:errorcluster)  [unwired: 1 in]
        n288 = call <vilib>:"Error Cluster From Error Code.vi"("error in (no error)"=w779, "error message (\"\")"=w782, "error code (0)"=1) -> ("error out"=w766:errorcluster)  [unwired: 6 in]
        n289 = Unbundle By Name(w766) -> ("source"=w767:string)
        n290 = Concatenate Strings(" [MAIN Loop] " ("error source (\" \")"), w767) -> (w769:string)
        n291 = Bundle By Name(cluster=w766, "source"=w769) -> (w765:errorcluster)
        n292 = call <vilib>:"Simple Error Handler.vi"("error in (no error)"=w765) -> ("error out"=w774:errorcluster)  [unwired: 4 in, 4 out]
        "UI ERROR" <- w774
        n293 = call <vilib>:"Clear Errors.vi"("error in (no error)"=w774) -> ("error out"=w771:errorcluster)  [unwired: 6 in]
        n294 = Flush Queue(queue=w772, error in (no error)=w771) -> (error out=w770:errorcluster)  [unwired: 2 out]
        n295 = Generate User Event "Generate\nUser Event"(user event=w773, event data cluster=w776, error in=w770) -> (error out=w775:errorcluster)  [unwired: 1 out]
      }
    }
    "MAIN Loop" <- w372
  }
  n296 = Unregister For Events(event registration refnum=w12, error in=w2) -> (error out=w1:errorcluster)
  n297 = call <vilib>:"Clear Errors.vi"("error in (no error)"=w1) -> ()  [unwired: 6 in, 1 out]
